vi "Day 12 - Part two.vi"() -> ()   [LabVIEW 2023]
panel:
  in  "input":string="abccccaaacaccccaaaaacccccccaaccccccccaaaaaaccccccaaaaaccccccccccaaaaaaaaacccccccaaaaaaaaaaaaaaccaaaaaccccccccccccaccacccccccccccccccccccccccccccccccccccccccaaaaaa\nabccaacaaaaaccaaaaacccccaaaaaccccccccaaaaaaccccccaaaaaacccccccccaaaaaaaaaaaaacccaaaaaaaaaaaaaaaaaaaaaccccccccccccaaaacccccccccccccccccccccccccccccccccccccccaaaaaa\nabccaaaaaaaaccaaaaaacccccaaaaaccccccaaaaaaaacccccaaaaaaccccccccccaaaaaaaaaaaacccaaaaaacaaaaaacaaaaaaaaccccccccccaaaaacccccaccccccccccccccccccaaacccccccccccccaaaaa\nabcccaaaaaccccccaaaacccccaaaaacccccaaaaaaaaaaccccaaaaaacccccccccaaaaaaaaaaaaaacaaaaaaaaaaaaaacaaaaaaaaccccccccc..."
  out "Visited":bool[][](array[boolean])
  out "Distance":u32
  out "E+Z":T1
  out "Intensity Graph":i32[][](graph)
  in  "test":bool
  in  "test input":string="Sabqponm\nabcryxxl\naccszExk\nacctuvwj\nabdefghi\n"
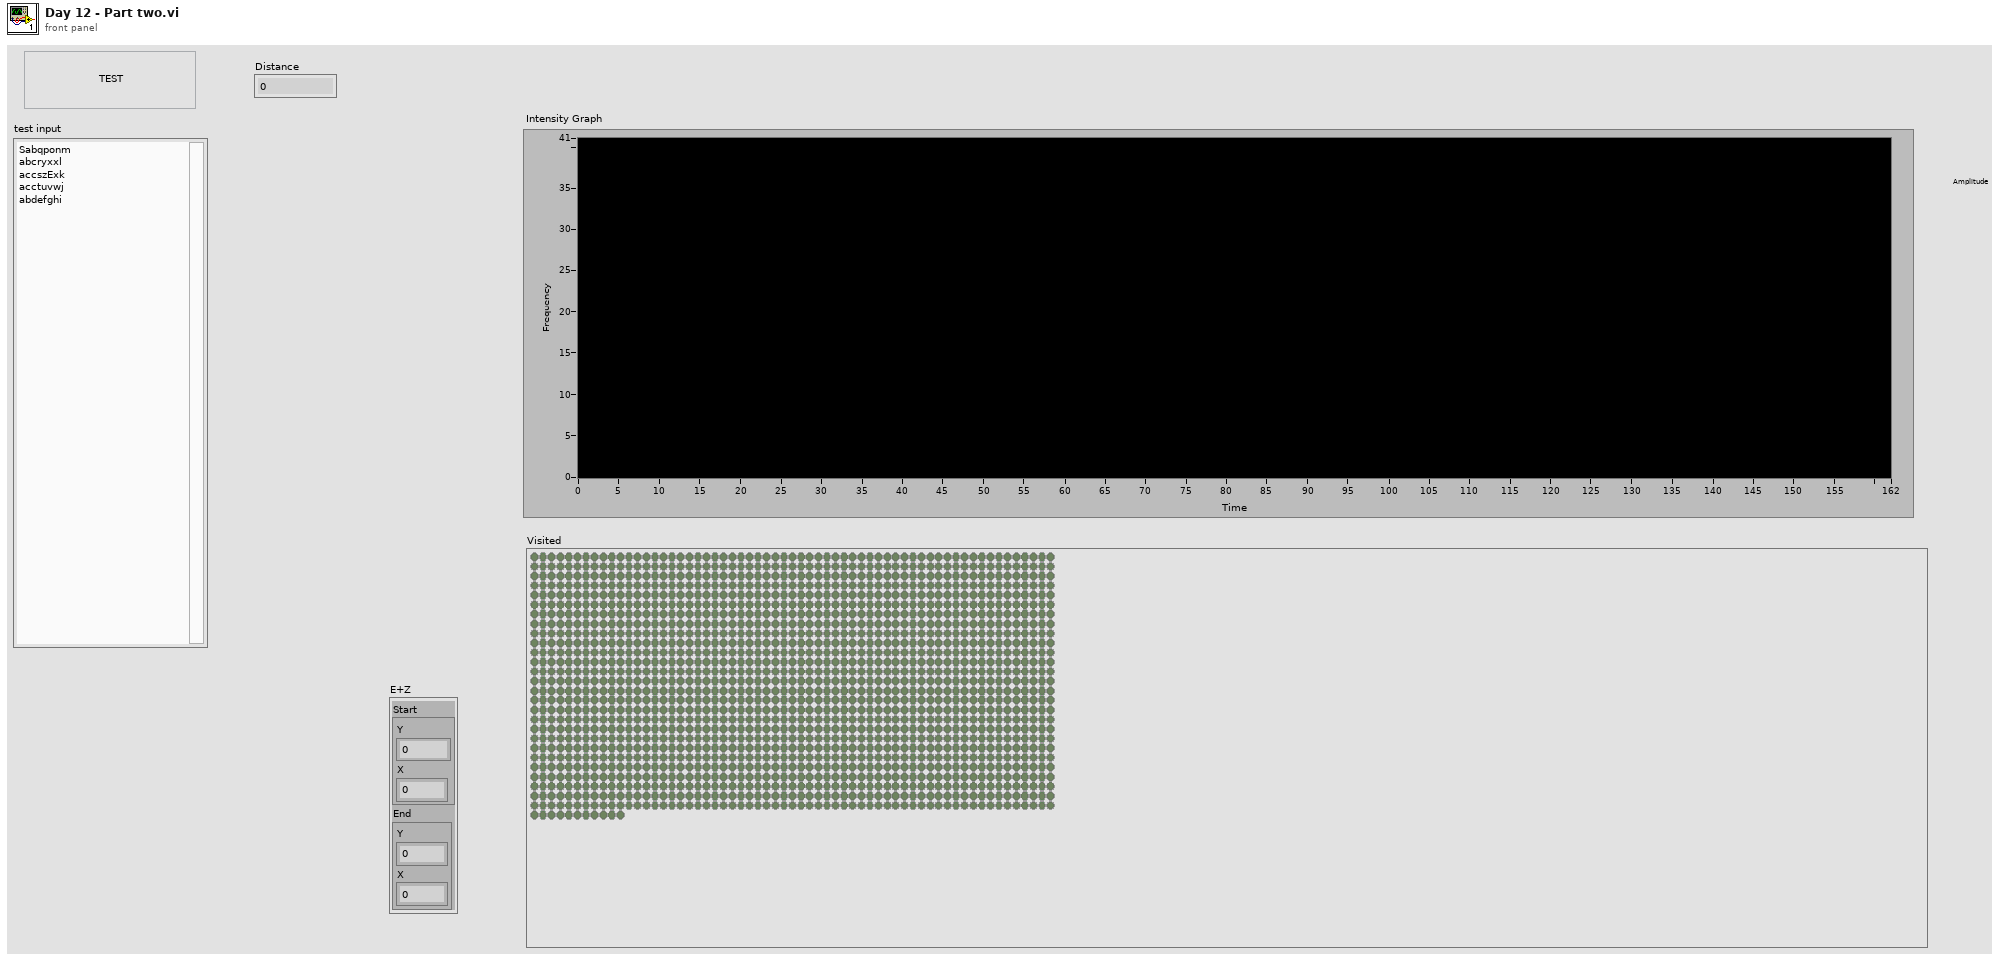
[diagram p1: front panel]
types:
  T1 = cluster{"Start":cluster{"Y":i32, "X":i32}, "End":cluster{"Y":i32, "X":i32}}
  T2 = cluster{"Distance":u32, "point":cluster{"Y":i32, "X":i32}}
  T3 = cluster{"Distance":u32, "point":cluster{"Y":i32, "X":i32}, "previus point":cluster{"Y":i32, "X":i32}, "Level":i32, "visited":bool}
  T4 = cluster{"Distance":u32, "point":cluster{"Y":i32, "X":i32}, "previus point":cluster{"Y":i32, "X":i32}, "Level":i32, "visited":bool}[][]
  T5 = cluster{"Distance":u32, "point":cluster{"Y":i32, "X":i32}}[]
  T6 = cluster{"Distance":u32, "Priority\nQueue":cluster{"Distance":u32, "point":cluster{"Y":i32, "X":i32}}}
  T7 = cluster{"Distance":u32, "Priority\nQueue":cluster{"Distance":u32, "point":cluster{"Y":i32, "X":i32}}}[]
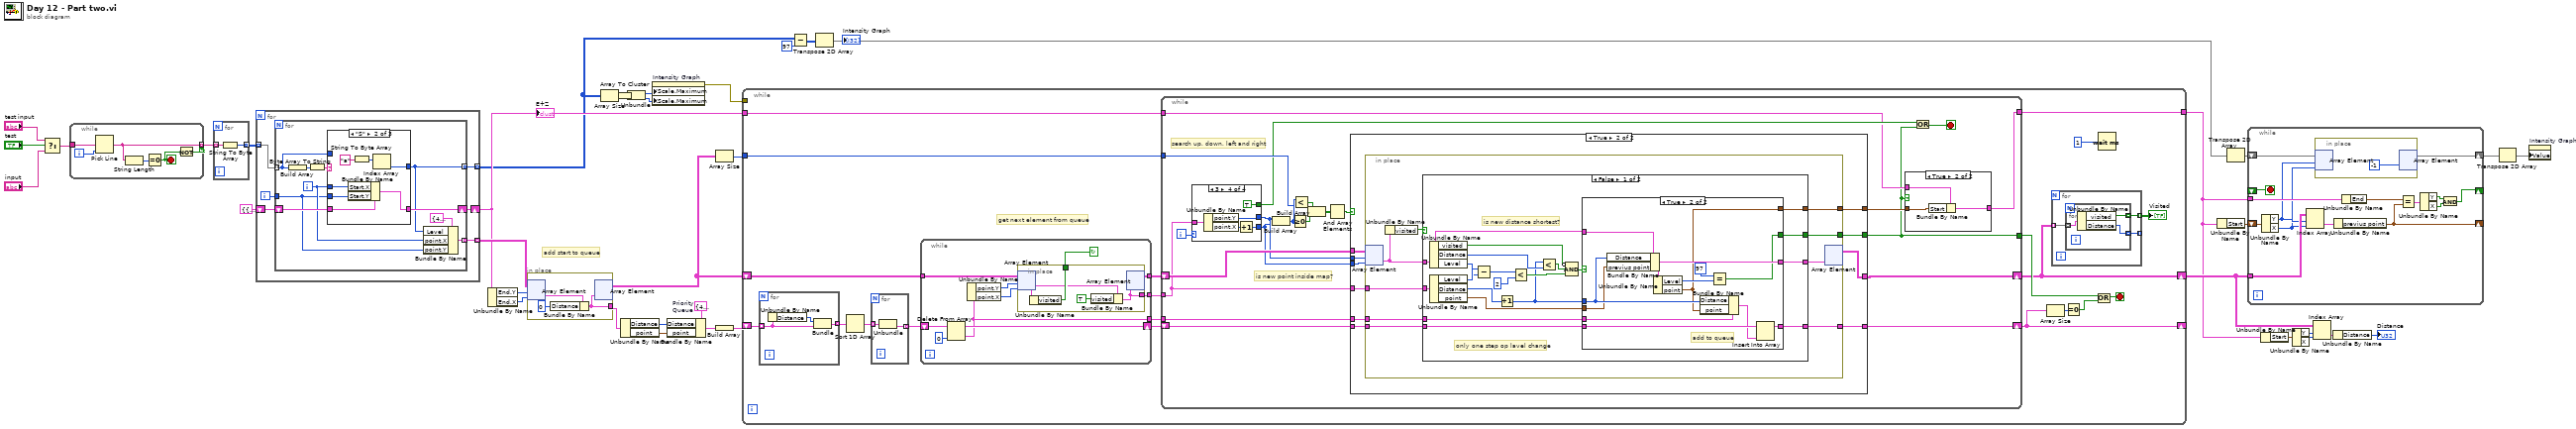
[diagram p0: block diagram]
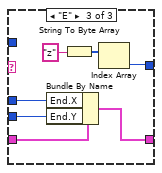
[diagram p3: hidden frame]
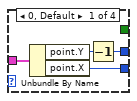
[diagram p8: hidden frame]
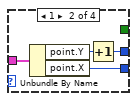
[diagram p9: hidden frame]
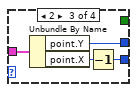
[diagram p10: hidden frame]
diagram:
  w27 = T2 {"Distance"=4294967295, "point"={"Y"=0, "X"=0}}  # Priority Queue
  # "add start to queue"
  n1 = Select(t="test input", s="test", f="input") -> (s? t:f=w38:string)
  n2 = while {
    tunnel: w38 -> [w43]
    tunnel: [w42] -> w35 mode=indexing if=w40
    i -> [w44]
    stop <- w41 stop-if-true
    n3 = Pick Line(multi-line string=w43, line index=w44) -> (output string=w42:string)  [unwired: 1 in]
    n4 = String Length(string=w42) -> (length=w45:i32)
    n5 = Equal To 0?(x=w45) -> (x = 0?=w41:bool)
    n6 = Not(x=w41) -> (.not. x?=w40:bool)
  }
  n7 = for {
    tunnel: w35 -> [w47] mode=indexing
    tunnel: [w46] -> w32 mode=indexing
    n8 = String To Byte Array(string=w47) -> (unsigned byte array=w46:u8[])
  }
  n9 = for {
    tunnel: w32 -> [w53] mode=indexing
    shift-right: [w50] -> w15
    shift-left: T1 {"Start"={"Y"=0, "X"=0}, "End"={"Y"=0, "X"=0}} -> [w52]
    tunnel: [w49] -> w8 mode=indexing
    tunnel: [w48] -> w29 mode=indexing
    i -> [w51]
    n10 = for {
      tunnel: w53 -> [w59] mode=indexing
      shift-right: [w60] -> w50
      shift-left: w52 -> [w61]
      tunnel: w51 -> [w55]
      tunnel: [w58] -> w49 mode=indexing
      tunnel: [w57] -> w48 mode=indexing
      i -> [w56]
      n11 = Build Array(w59) -> (w63:u8[])
      n12 = Byte Array To String(unsigned byte array=w63) -> (string=w62:string)
      n13 = case shown="\"S\"" w62 {
        tunnel: w61 -> [w65 w72 w79]
        tunnel: [w65 w71 w78] -> w60
        tunnel: w55 -> [_ w69 w77]
        tunnel: w56 -> [_ w70 w76]
        tunnel: [w64 w66 w73] -> w58
        tunnel: w59 -> [w64 _ _]
        frame "False", Default {
        }
        frame "S" {
          n14 = Bundle By Name(cluster=w72, "Start.X"=w70, "Start.Y"=w69) -> (w71:T1)
          n15 = String To Byte Array(string="a") -> (unsigned byte array=w67:u8[])
          n16 = Index Array(array=w67) -> (element=w66:u8)  [unwired: 1 in]
        }
        frame "E" {
          n17 = Bundle By Name(cluster=w79, "End.X"=w76, "End.Y"=w77) -> (w78:T1)
          n18 = String To Byte Array(string="z") -> (unsigned byte array=w74:u8[])
          n19 = Index Array(array=w74) -> (element=w73:u8)  [unwired: 1 in]
        }
      }
      n20 = Bundle By Name(cluster=T3 {"Distance"=4294967295, "point"={"Y"=0, "X"=0}, "previus point"={"Y"=-1, "X"=-1}, "Level"=0, "visited"=FALSE}, "Level"=w58, "point.X"=w56, "point.Y"=w55) -> (w57:T3)
    }
  }
  "E+Z" <- w15
  n21 = Unbundle By Name(w15) -> ("End.Y"=w30:i32, "End.X"=w28:i32)
  n22 = in-place {
    in-place-border: [w80] -> w26
    n23 = in-place-array #1(w29, w30, w28) -> (w82:T3)
    n24 = Bundle By Name(cluster=w82, "Distance"=u32 0) -> (w80:T3)
    n25 = in-place-array #1(w80) -> (w21:T4)  [unwired: 2 out]
  }
  n26 = Array Size(array=w8) -> (size(s)=w7:i32[])
  n27 = Array To Cluster(array=w7) -> (cluster=w6:cluster{"[0]":i32, "[1]":i32})
  n28 = Unbundle By Name(w26) -> ("Distance"=w24:u32, "point"=w25:cluster{"Y":i32, "X":i32})
  n29 = Unbundle(w6) -> ("[0]"=w5:i32, "[1]"=w4:i32)
  n30 = property on="Intensity Graph" class="IntGraph (strict)"("YScale.Maximum"=w5, "XScale.Maximum"=w4) -> (error out=w3:errorcluster)  [unwired: 2 in, 1 out]
  n31 = Bundle By Name(cluster=w27, "Distance"=w24, "point"=w25) -> (w23:T2)
  n32 = Build Array(w23) -> (w22:T5)
  n33 = Array Size(array=w21) -> (size(s)=w20:i32[])
  n34 = while {
    shift-right: [w89] -> _
    shift-left: w22 -> [w102]
    shift-right: [w91] -> w13
    shift-left: w21 -> [w98]
    tunnel: w20 -> [w94]
    tunnel: w15 -> [w84]
    tunnel: [w83] -> w2
    tunnel: w3 -> [_]
    stop <- w87 stop-if-true
    # "get next element from queue"
    n35 = for {
      tunnel: w102 -> [w120] mode=indexing
      tunnel: [w119] -> w101 mode=indexing
      n36 = Unbundle By Name(w120) -> ("Distance"=w121:u32)
      n37 = Bundle("Distance"=w121, "Priority\nQueue"=w120) -> (w119:T6)  [unwired: 1 in]
    }
    n38 = Sort 1D Array(array=w101) -> (sorted array=w100:T7)
    n39 = for {
      tunnel: w100 -> [w118] mode=indexing
      tunnel: [w117] -> w99 mode=indexing
      n40 = Unbundle(w118) -> ("Priority\nQueue"=w117:T2)  [unwired: 1 out]
    }
    n41 = while {
      shift-right: [w112] -> w95
      shift-left: w99 -> [w104]
      tunnel: w98 -> [w110]
      tunnel: [w105] -> w96
      tunnel: [w109] -> w97
      tunnel: [w111] -> w93
      stop <- w106 continue-if-true
      n42 = Delete From Array(array=w104, index=0) -> (deleted portion=w111:T2, array with subset deleted=w112:T5)  [unwired: 1 in]
      n43 = Unbundle By Name(w111) -> ("point.Y"=w108:i32, "point.X"=w107:i32)
      n44 = in-place {
        in-place-border: [w116] -> w106
        in-place-border: [w113] -> w105
        n45 = in-place-array #2(w110, w108, w107) -> (w115:T3)
        n46 = Unbundle By Name(w115) -> ("visited"=w116:bool)
        n47 = Bundle By Name(cluster=w115, "visited"=TRUE) -> (w113:T3)
        n48 = in-place-array #2(w113) -> (w109:T4)  [unwired: 2 out]
      }
    }
    n49 = while {
      tunnel: w96 -> [w127]
      tunnel: w94 -> [w137]
      tunnel: w93 -> [w130]
      tunnel: [w122] -> w92
      shift-right: [w131] -> w89
      shift-left: w95 -> [w132]
      shift-right: [w129] -> w91
      shift-left: w97 -> [w135]
      tunnel: w84 -> [w125]
      tunnel: [w124] -> w83
      i -> [w142]
      stop <- w123 stop-if-true
      # "search up, down, left and right"
      # "is new point inside map?"
      n50 = case shown="3" w142 {
        tunnel: w127 -> [w207 w211 w215 w220]
        tunnel: [w204 w208 w213 w218] -> w134
        tunnel: [w205 w209 w212 w217] -> w133
        tunnel: [_ _ _ TRUE] -> w128
        frame 0, Default {
          n51 = Unbundle By Name(w207) -> ("point.Y"=w206:i32, "point.X"=w205:i32)
          n52 = Decrement(x=w206) -> (x-1=w204:i32)
        }
        frame 1 {
          n53 = Unbundle By Name(w211) -> ("point.Y"=w210:i32, "point.X"=w209:i32)
          n54 = Increment(x=w210) -> (x+1=w208:i32)
        }
        frame 2 {
          n55 = Unbundle By Name(w215) -> ("point.Y"=w213:i32, "point.X"=w214:i32)
          n56 = Decrement(x=w214) -> (x-1=w212:i32)
        }
        frame 3 {
          n57 = Unbundle By Name(w220) -> ("point.Y"=w218:i32, "point.X"=w219:i32)
          n58 = Increment(x=w219) -> (x+1=w217:i32)
        }
      }
      n59 = Build Array(w134, w133) -> (w141:i32[])
      n60 = Greater Or Equal To 0?(x=w141) -> (x >= 0?=w139:bool[])
      n61 = Less?(x=w141, y=w137) -> (x < y?=w140:bool[])
      n62 = Build Array(w140, w139) -> (w138:bool[][])
      n63 = And Array Elements(Boolean array=w138) -> (logical AND=w136:bool)
      n64 = case shown="True" w136 {
        tunnel: w135 -> [w147 w158]
        tunnel: w134 -> [_ w157]
        tunnel: w133 -> [_ w156]
        tunnel: w127 -> [_ w155]
        tunnel: w132 -> [w148 w154]
        tunnel: [w148 w153] -> w131
        tunnel: w130 -> [_ w152]
        tunnel: [w147 w151] -> w129
        tunnel: [_ w150] -> w122
        tunnel: [_ w149] -> w126
        frame False {
        }
        frame True {
          n65 = in-place {
            in-place-border: w155 -> [w165]
            in-place-border: w154 -> [w167]
            in-place-border: [w166] -> w153
            in-place-border: w152 -> [w164]
            in-place-border: [w163] -> w150
            in-place-border: [w159] -> w149
            n66 = in-place-array #3(w158, w157, w156) -> (w162:T3)
            n67 = Unbundle By Name(w162) -> ("visited"=w161:bool)
            n68 = case shown="False" w161 {
              tunnel: w162 -> [w185 w203]
              tunnel: [w182 w203] -> w160
              tunnel: w167 -> [w181 w202]
              tunnel: [w180 w202] -> w166
              tunnel: w165 -> [w179 _]
              tunnel: w164 -> [w178 _]
              tunnel: [w173 _] -> w163
              tunnel: [w168 _] -> w159
              frame False {
                # "is new distance shortest?"
                # "only one step op lavel change"
                n69 = Unbundle By Name(w185) -> ("visited"=w172:bool, "Distance"=w175:u32, "Level"=w171:i32)
                n70 = Unbundle By Name(w179) -> ("Level"=w187:i32, "Distance"=w170:u32, "point"=w183:cluster{"Y":i32, "X":i32})
                n71 = Subtract(x=w187, y=w171) -> (x-y=w169:i32)
                n72 = Increment(x=w170) -> (x+1=w174:u32)
                n73 = Less?(x=w169, y=2) -> (x < y?=w184:bool)
                n74 = Less?(x=w174, y=w175) -> (x < y?=w176:bool)
                n75 = Compound Arithmetic op=AND(invert w172, w176, w184) -> (w177:bool)
                n76 = case shown="True" w177 {
                  tunnel: w185 -> [w189 w201]
                  tunnel: w174 -> [_ w200]
                  tunnel: w183 -> [_ w199]
                  tunnel: [w189 w195] -> w182
                  tunnel: w181 -> [w188 w198]
                  tunnel: [w188 w197] -> w180
                  tunnel: w178 -> [_ w196]
                  tunnel: [_ w191] -> w173
                  tunnel: [_ w190] -> w168
                  frame False {
                  }
                  frame True {
                    # "add to queue"
                    n77 = Bundle By Name(cluster=w201, "Distance"=w200, "previus point"=w199) -> (w195:T3)
                    n78 = Unbundle By Name(w195) -> ("Level"=w193:i32, "point"=w190:cluster{"Y":i32, "X":i32})
                    n79 = Bundle By Name(cluster=w196, "Distance"=w200, "point"=w190) -> (w194:T2)
                    n80 = Equal?(x=97, y=w193) -> (x = y?=w191:bool)
                    n81 = Insert Into Array(array=w198, new element=w194) -> (w197:T5)  [unwired: 1 in]
                  }
                }
              }
              frame True {
              }
            }
            n82 = in-place-array #3(w160) -> (w151:T4)  [unwired: 2 out]
          }
        }
      }
      n83 = case shown="True" w122 {
        tunnel: w126 -> [_ w146]
        tunnel: w125 -> [w143 w145]
        tunnel: [w143 w144] -> w124
        frame False {
        }
        frame True {
          n84 = Bundle By Name(cluster=w145, "Start"=w146) -> (w144:T1)
        }
      }
      n85 = Or(x=w128, y=w122) -> (x .or. y?=w123:bool)
    }
    n86 = Array Size(array=w89) -> (size(s)=w88:i32)
    n87 = for {
      tunnel: w91 -> [w223] mode=indexing
      tunnel: [w222] -> w90 mode=indexing
      tunnel: [w221] -> _ mode=indexing
      n88 = for {
        tunnel: w223 -> [w226] mode=indexing
        tunnel: [w225] -> w222 mode=indexing
        tunnel: [w224] -> w221 mode=indexing
        n89 = Unbundle By Name(w226) -> ("visited"=w225:bool, "Distance"=w224:u32)
      }
    }
    "Visited" <- w90
    n90 = Equal To 0?(x=w88) -> (x = 0?=w86:bool)
    n91 = Or(x=w92, y=w86) -> (x .or. y?=w87:bool)
    n92 = Wait (ms)(milliseconds to wait=u32 1) -> ()  [unwired: 1 out]
  }
  n93 = Subtract(x=w8, y=97 ("Numeric")) -> (x-y=w31:i32[][])
  n94 = Transpose 2D Array(2D array=w31) -> (transposed array=w12:i32[][])
  "Intensity Graph" <- w12
  n95 = Unbundle By Name(w2) -> ("Start"=w1:cluster{"Y":i32, "X":i32})
  n96 = Transpose 2D Array(2D array=w12) -> (transposed array=w10:i32[][])
  n97 = while {
    tunnel: w13 -> [w241]
    shift-right: [w233] -> _
    shift-left: w1 -> [w240]
    tunnel: w2 -> [w235]
    shift-right: [w231] -> w11
    shift-left: w10 -> [w232]
    shift-right: [w228] -> _
    shift-left: _ -> [w227]
    stop <- w227 stop-if-true
    n98 = Unbundle By Name(w240) -> ("Y"=w230:i32, "X"=w229:i32)
    n99 = Index Array(array=w241, index (row)=w230, index (col)=w229) -> (element=w239:T3)
    n100 = in-place {
      n101 = in-place-array #4(w232, w230, w229) -> ()  [unwired: 1 out]
      n102 = in-place-array #4(-1 ("x")) -> (w231:i32[][])  [unwired: 2 out]
    }
    n103 = Unbundle By Name(w239) -> ("previus point"=w233:cluster{"Y":i32, "X":i32})
    n104 = Unbundle By Name(w235) -> ("End"=w234:cluster{"Y":i32, "X":i32})
    n105 = Equal?(x=w234, y=w233) -> (x = y?=w236:cluster{"Y":bool, "X":bool})
    n106 = Unbundle By Name(w236) -> ("Y"=w237:bool, "X"=w238:bool)
    n107 = And(x=w237, y=w238) -> (x .and. y?=w228:bool)
  }
  n108 = Unbundle By Name(w2) -> ("Start"=w14:cluster{"Y":i32, "X":i32})
  n109 = Unbundle By Name(w14) -> ("Y"=w19:i32, "X"=w18:i32)
  n110 = Index Array(array=w13, index (row)=w19, index (col)=w18) -> (element=w17:T3)
  n111 = Unbundle By Name(w17) -> ("Distance"=→"Distance":u32)
  n112 = Transpose 2D Array(2D array=w11) -> (transposed array=w9:i32[][])
  n113 = property on="Intensity Graph" class="IntGraph (strict)"("Value"=w9) -> ()  [unwired: 2 in, 2 out]
